vi "test_tcp_server.vi"() -> ()   [LabVIEW 2013]
uses:
  response.ctl
  driver_status.ctl
  Driver/RemoteConnection/RemoteReferences.ctl
  Driver/TcpServerDriver/TcpServerDriver.lvclass
  global_stop.vi
  Driver/RemoteConnection/RemoteConnection.lvclass
panel:
  in  "Output delay delta":dbl(slide) scale=0.0..6.0
  in  "Output delay":dbl(slide) scale=0.0..6.0
  in  "b":fxp<+/-,16,2>
  in  "a":fxp<+/-,16,2>
  in  "fm":dbl
  out "error out":errorcluster
  in  "stop":bool
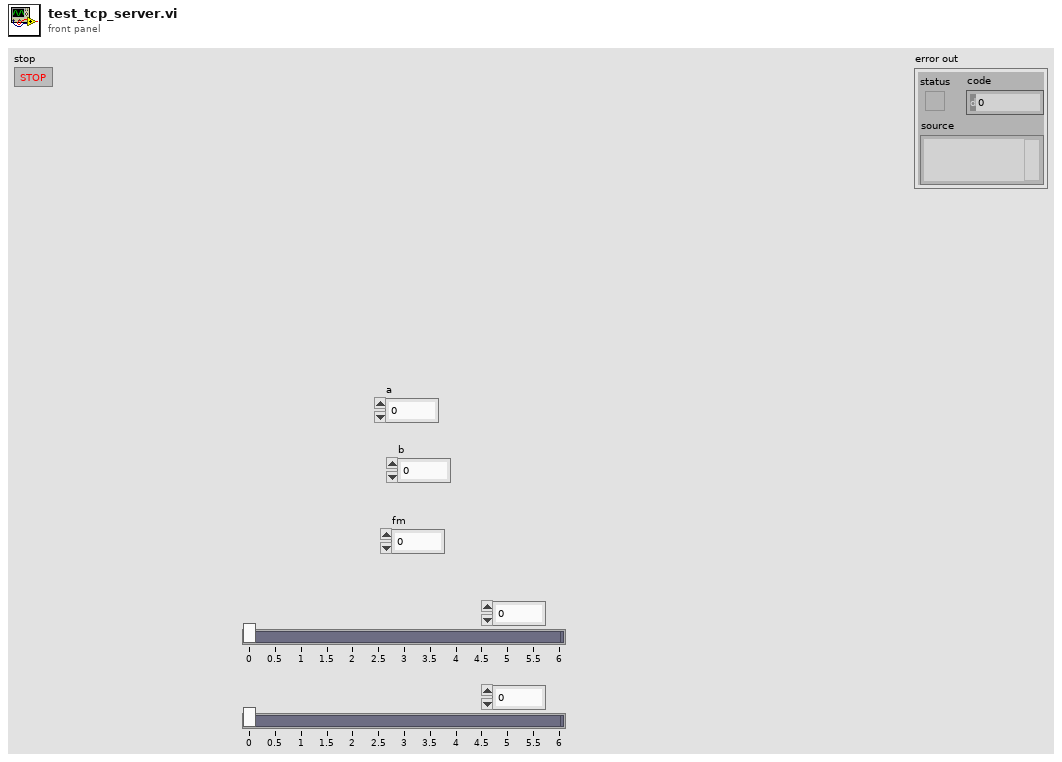
[diagram p1: front panel]
types:
  T1 = typedef "RemoteConnection.lvclass/RemoteReferences.ctl" = cluster{"a":refnum<vi>, "b":refnum<vi>, "fm":refnum<vi>, "Output delay":refnum<vi>, "Output delay delta":refnum<vi>}
  T2 = typedef "response.ctl" = cluster{"driver status":T3, "Sender":string, "Type":i32, "Variant":variant}
  T3 = typedef "driver_status.ctl" = enum16{"Normal", "Startup", "Connection lost", "Reconnected", "Timeout", "Idle", "Busy"}
  T4 = typedef "message_queue.ctl" = refnum<queue>
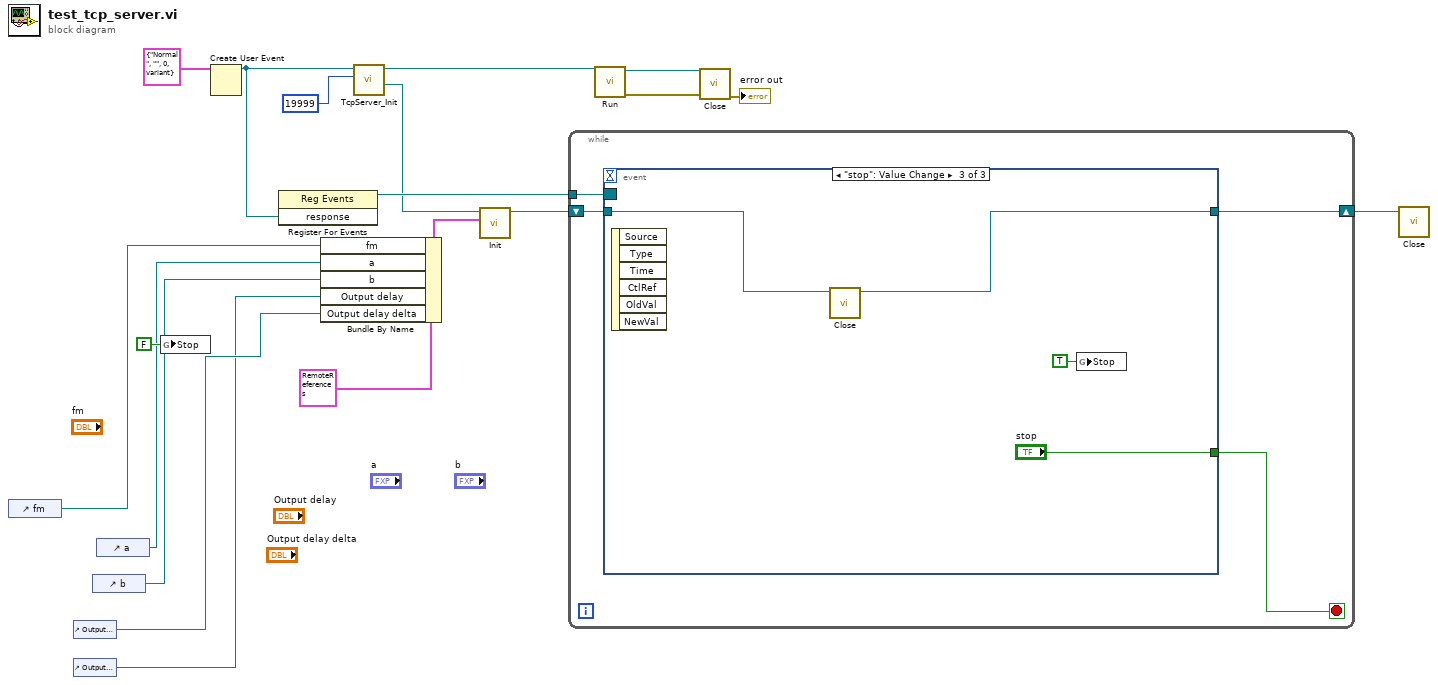
[diagram p0: block diagram]
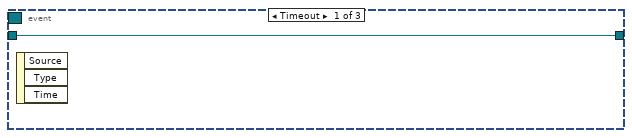
[diagram p2: hidden frame]
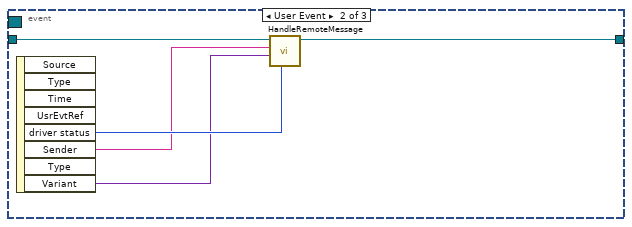
[diagram p3: hidden frame]
diagram:
  n1 = control-ref of="fm"() -> (w8:refnum<vi>)
  n2 = control-ref of="Output delay delta"() -> (w2:refnum<vi>)
  n3 = control-ref of="Output delay"() -> (w1:refnum<vi>)
  n4 = control-ref of="b"() -> (w3:refnum<vi>)
  n5 = control-ref of="a"() -> (w4:refnum<vi>)
  n6 = global write "global_stop.vi" "Stop"(FALSE ("Stop")) -> ()
  n7 = Create User Event(user event datatype=T2 {"driver status"=enum."Normal", "Sender"="", "Type"=0, "Variant"=variant} ("response")) -> (user event=w17:refnum<user-event>)  [unwired: 1 in, 1 out]
  n8 = register-events(w17) -> (reference out=w16:refnum<event-registration>)  [unwired: 2 in, 1 out]
  n9 = Bundle By Name(cluster=T1 {"a"=refnum, "b"=refnum, "fm"=refnum, "Output delay"=refnum, "Output delay delta"=refnum} ("refs"), "fm"=w8, "a"=w4, "b"=w3, "Output delay"=w1, "Output delay delta"=w2) -> (w7:T1)
  n10 = call "TcpServer_Init.vi"("local port"=u16 19999, "response event"=w17) -> ("Message queue"=w10:T4, "TcpServerDriver"=w15:refnum<class "TcpServerDriver.lvclass">)  [unwired: 8 in]
  n11 = call "Init.vi"("refs"=w7, "server queue"=w10) -> ("RemoteConnection"=w6:refnum<class "RemoteConnection.lvclass">)  [unwired: 9 in]
  n12 = while {
    tunnel: w16 -> [w23]
    shift-right: [w20] -> w5
    shift-left: w6 -> [w21]
    stop <- w22 stop-if-true
    n13 = event shown="[2] \"stop\": Value Change" {
      selector: w23 -> [_ _ _]
      dyn-events: _ -> [_ _ _]
      timeout: _ -> [_ _ _]
      tunnel: [_ _ "stop"] -> w22
      tunnel: w21 -> [w24 w29 w31]
      tunnel: [w24 w25 w30] -> w20
      event Timeout {
        n14 = event-data() -> ()  [unwired: 1 in, 3 out]
      }
      event User Event {
        n15 = event-data() -> ("driver status"=w28:T3, "Sender"=w27:string, "Variant"=w26:variant)  [unwired: 1 in, 5 out]
        n16 = call "HandleRemoteMessage.vi"("driver status"=w28, "Message data"=w26, "Sender"=w27, "RemoteConnection in"=w29) -> ("RemoteConnection out"=w25:refnum<class "RemoteConnection.lvclass">)  [unwired: 6 in, 1 out]
      }
      event "stop": Value Change {
        n17 = event-data() -> ()  [unwired: 1 in, 6 out]
        n18 = call "Close.vi"("RemoteConnection in"=w31) -> ("RemoteConnection out"=w30:refnum<class "RemoteConnection.lvclass">)  [unwired: 9 in, 1 out]
        n19 = global write "global_stop.vi" "Stop"(TRUE ("Stop")) -> ()
      }
    }
  }
  n20 = call-dynamic "Run.vi"("BaseDriver in"=w15) -> ("error out"=w13:errorcluster, "BaseDriver out"=w14:refnum<class "TcpServerDriver.lvclass">)  [unwired: 9 in]
  n21 = call-dynamic "Close.vi"("error in (no error)"=w13, "BaseDriver in"=w14) -> ("error out"=→"error out":errorcluster)  [unwired: 8 in, 1 out]
  n22 = call "Close.vi"("RemoteConnection in"=w5) -> ()  [unwired: 9 in, 2 out]
